vi "TestFlowID - Read.vi"(8 "error in (no error)":errorcluster, 11 "Globals in":refnum<class "TSM Context Data Access.lvclass">) -> (0 "error out":errorcluster, 2 "TestFlowID":string, 3 "Globals out":refnum<class "TSM Context Data Access.lvclass">)   [LabVIEW 2019, in "TSM Context Data Access.lvclass"]
uses:
  TSM Context Data Access.lvclass
  TSM Context Data Access.lvclass/TSM Context Data Access.ctl
  <vilib>/NI_TestStand_SemiconductorModule/NI_TestStand_Semiconductor_Module.lvlibp
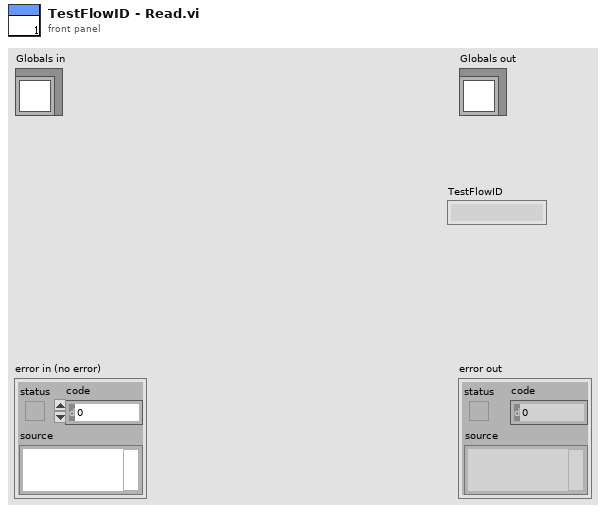
[diagram p1: front panel]
types:
  T1 = typedef "NI_TestStand_Semiconductor_Module.lvlibp/SemiconductorModuleContext.ctl" = refnum<k7>
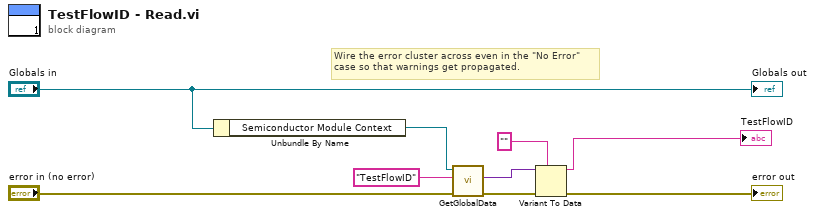
[diagram p0: block diagram]
diagram:
  # "Wire the error cluster across even in the \"No Error\"\ncase so that warnings get propagated."
  n1 = Unbundle By Name("Globals in") -> ("Semiconductor Module Context"=w5:T1)
  n2 = call <vilib>:"GetGlobalData.vi"("error in (no error)"="error in (no error)", "Data Id"="TestFlowID", "Semiconductor Module Context"=w5) -> ("error out"=w1:errorcluster, "Data"=w3:variant)  [unwired: 6 in, 1 out]
  n3 = Variant To Data(error in=w1, type="", Variant=w3) -> (data=→"TestFlowID":string, error out=→"error out":errorcluster)
  "Globals out" <- "Globals in"
